vi "Initialize.vi"(0 "DashboardServer in":refnum<class "Dashboard Server.lvclass">, 5 "error in (no error)":errorcluster) -> (14 "DashboardServer out":refnum<class "Dashboard Server.lvclass">, 19 "error out":errorcluster)   [LabVIEW 2016, in "Dashboard Server.lvclass"]
uses:
  Dashboard Server.lvclass
  Dashboard Server.lvclass/Dashboard Server.ctl
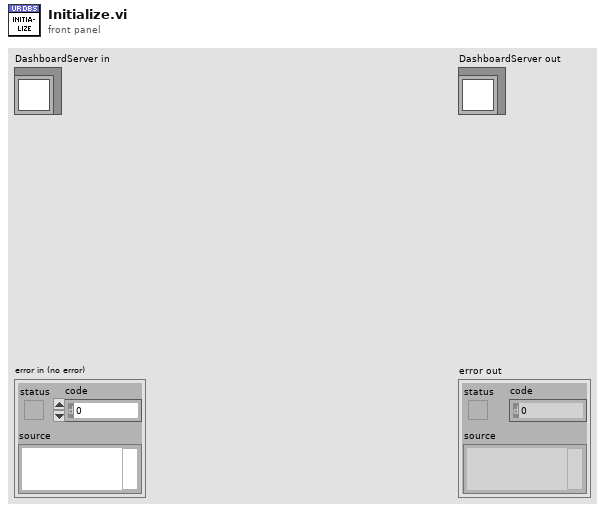
[diagram p1: front panel]
types:
  T1 = typedef "Semaphore RefNum" = refnum<k1>
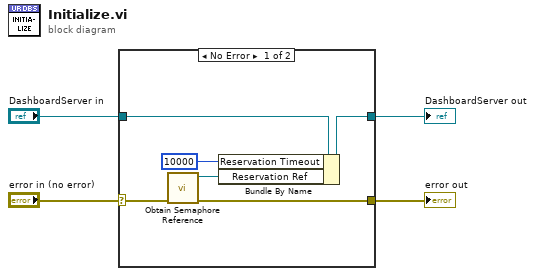
[diagram p0: block diagram]
diagram:
  n1 = case shown="No Error" "error in (no error)" {
    selector: "error in (no error)" -> [w10 w12]
    tunnel: [w6 w12] -> w3
    tunnel: [w7 w11] -> w1
    tunnel: "DashboardServer in" -> [w9 w11]
    frame No Error {
      n2 = call <vilib>:"Obtain Semaphore Reference.vi"("error in (no error)"=w10) -> ("error out"=w6:errorcluster, "semaphore"=w8:T1)  [unwired: 4 in, 1 out]
      n3 = Bundle By Name(cluster=w9, "Reservation Timeout"=10000 ("reservationTimeout"), "Reservation Ref"=w8) -> (w7:refnum<class "Dashboard Server.lvclass">)
    }
    frame Error {
    }
  }
  "error out" <- w3
  "DashboardServer out" <- w1
